vi "GyroTurn.vi"(10 "Wheel Velocity":dbl, 11 "Angle":dbl) -> ()   [LabVIEW 2012]
uses:
  Auto_Conf.vi
  <vilib>/Rock Robotics/WPI/RobotDrive/WPI_RobotDriveGetSetRefNum.vi
  <vilib>/Rock Robotics/WPI/RobotDrive/WPI_RobotDriveMecanumDrive_Cartesian.vi
panel:
  in  "Overshoot Neg":dbl=-6.0
  in  "Overshoot":dbl=16.0
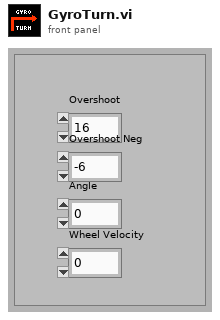
[diagram p1: front panel]
types:
  T1 = typedef "WPI_GyroDevRef.ctl" = cluster{"DevStatus":errorcluster, "Analog Module":T2, "Analog Channel":T3, "Offset":dbl, "Gain (VoltsPerDegree/Second)":dbl}
  T2 = typedef "FPGA_TypedefAnalogModule.ctl" = enum16{"Analog Module 1", "Analog Module 2"}
  T3 = typedef "FPGA_AIChannel.ctl" = enum8{"AI 1", "AI 2", "AI 3", "AI 4", "AI 5", "AI 6", "AI 7", "AI 8", "Invalid"}
  T4 = typedef "WPI_RobotDriveDevRef.ctl" = cluster{"DevStatus":errorcluster, "Motors[]":T5[], "Square Inputs":bool, "Max Output":dbl, "Isochronous":bool}
  T5 = typedef "WPI_MotorControlDeviceRef.ctl" = cluster{"DeviceStatus":errorcluster, "Type":enum16{"PWM", "CAN"}, "PWM":cluster{"Digital Module":T6, "PWM Channel":T7, "DeadBand":T8}, "CAN":cluster{"Device Number":u8, "Control Mode":T9, "Semaphore":T10, "Max Vout":dbl}, "Invert":bool, "TransformRef":T11, "InvTransformRef":T11}
  T6 = typedef "FPGA_TypedefDigitalModule.ctl" = enum16{"Digital Module 1", "Digital Module 2"}
  T7 = typedef "FPGA_DIOPWMChannel.ctl" = enum8{"PWM 1", "PWM 2", "PWM 3", "PWM 4", "PWM 5", "PWM 6", "PWM 7", "PWM 8", "PWM 9", "PWM 10", "Invalid"}
  T8 = typedef "WPI_PWMDeadband.ctl" = cluster{"Name":string, "maxPositivePwm":i32, "minPositivePwm":i32, "centerPwm":i32, "maxNegativePwm":i32, "minNegativePwm":i32, "angularRange":u16}
  T9 = typedef "WPI_CANJaguar_ControlMode.ctl" = enum8{"Percent VBus", "Current", "Speed", "Position", "Voltage"}
  T10 = typedef "Semaphore RefNum" = refnum<k1>
  T11 = typedef "WPI_PWMTransform_ConPane.ctl" = refnum<vi>
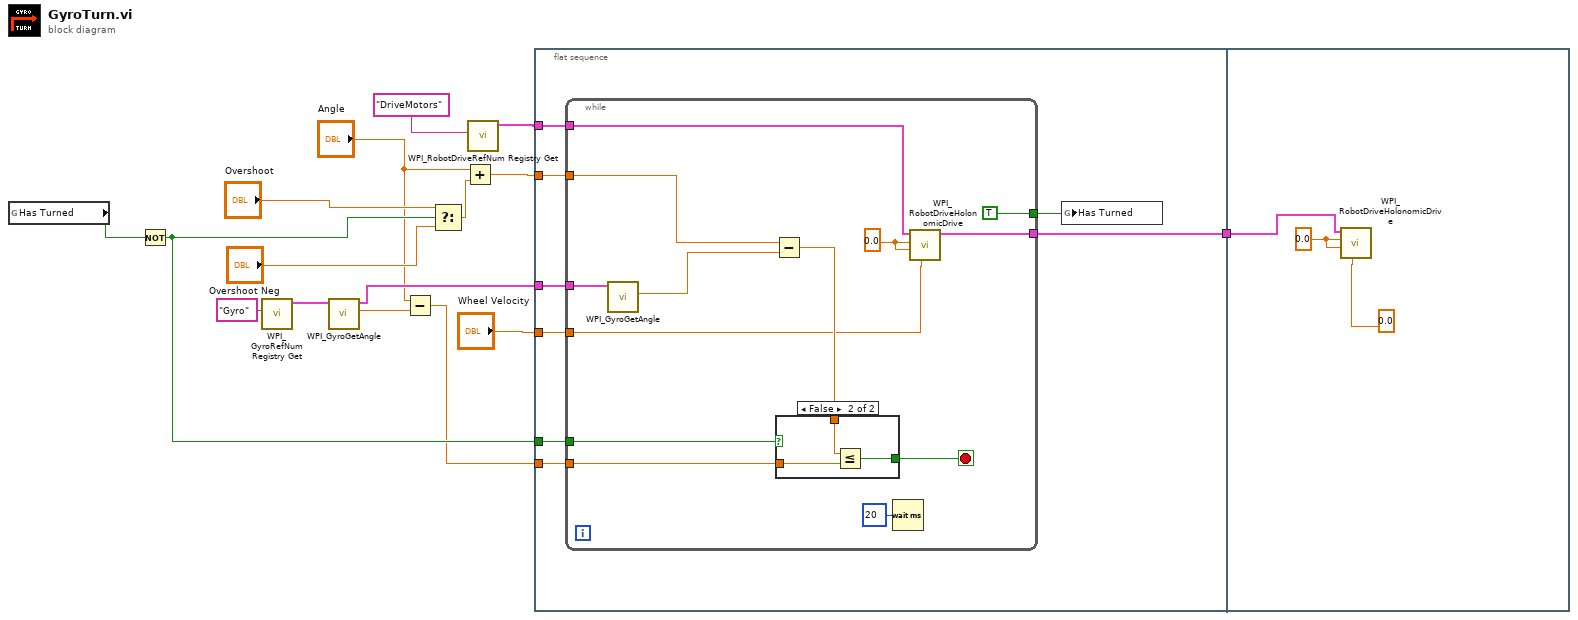
[diagram p0: block diagram]
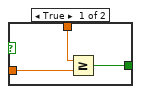
[diagram p2: hidden frame]
diagram:
  n1 = global read "Auto_Conf.vi" "Has Turned"() -> (w7:bool)
  n2 = Not(x=w7) -> (.not. x?=w6:bool)
  n3 = call <vilib>:"WPI_GyroRefNum Registry Get.vi"("refnum name"="Gyro") -> ("GyroDevRef"=w9:T1)  [unwired: 1 in, 9 out]
  n4 = call <vilib>:"WPI_GyroGetAngle.vi"("GyroDevRef"=w9) -> ("Angle"=w10:dbl, "GyroDevRef"=w8:T1)  [unwired: 1 in, 8 out]
  n5 = Subtract(x="Angle", y=w10) -> (x-y=w4:dbl)
  n6 = Select(t="Overshoot", s=w6, f="Overshoot Neg") -> (s? t:f=w12:dbl)
  n7 = Add(x="Angle", y=w12) -> (x+y=w14:dbl)
  n8 = call <vilib>:"WPI_RobotDriveRefNum Registry Get.vi"("refnum name"="DriveMotors") -> ("RobotDriveDevRef"=w3:T4)  [unwired: 9 in, 1 out]
  n9 = flat-sequence {
    tunnel: "Wheel Velocity" -> [w24]
    tunnel: w14 -> [w23]
    tunnel: w8 -> [w22]
    tunnel: w6 -> [w20]
    tunnel: w4 -> [w19]
    tunnel: w3 -> [w18]
    tunnel: [w17] -> w1
    tunnel: w1 -> [w44]
    frame #0 {
      n10 = while {
        tunnel: w24 -> [w26]
        tunnel: w23 -> [w29]
        tunnel: w22 -> [w35]
        tunnel: [TRUE ("Has Turned")] -> w21
        tunnel: w20 -> [w32]
        tunnel: w19 -> [w31]
        tunnel: w18 -> [w30]
        tunnel: [w25] -> w17
        stop <- w37 stop-if-true
        w27 = 0.0 ("Magnitude")
        n11 = call <vilib>:"WPI_GyroGetAngle.vi"("GyroDevRef"=w35) -> ("Angle"=w34:dbl)  [unwired: 1 in, 9 out]
        n12 = Subtract(x=w29, y=w34) -> (x-y=w28:dbl)
        n13 = case shown="False" w32 {
          tunnel: [w40 w43] -> w37
          tunnel: w28 -> [w39 w42]
          tunnel: w31 -> [w38 w41]
          frame True {
            n14 = Greater Or Equal?(x=w39, y=w38) -> (x >= y?=w40:bool)
          }
          frame False {
            n15 = Less Or Equal?(x=w42, y=w41) -> (x <= y?=w43:bool)
          }
        }
        n16 = Wait (ms)(milliseconds to wait=u32 20) -> ()  [unwired: 1 out]
        n17 = call-poly <vilib>:"WPI_RobotDriveHolonomicDrive.vi"("Rotation"=w26, "Y"=w27, "X"=w27, "RobotDriveDevRef"=w30) -> ("RobotDriveDevRef"=w25:T4)  [unwired: 5 in, 2 out]
      }
      n18 = global write "Auto_Conf.vi" "Has Turned"(w21) -> ()
    }
    frame #1 {
      w46 = 0.0 ("Magnitude")
      n19 = call-poly <vilib>:"WPI_RobotDriveHolonomicDrive.vi"("Rotation"=0.0, "Y"=w46, "X"=w46, "RobotDriveDevRef"=w44) -> ()  [unwired: 5 in, 3 out]
    }
  }
